vi "Get Focus.vi"(8 "error in":errorcluster, 10 "Start Z":dbl, 11 "CameraTool Class In":refnum<class "CameraTool Class.lvclass">) -> (0 "error out":errorcluster, 2 "focus height":sgl, 3 "CameraTool Class Out":refnum<class "CameraTool Class.lvclass">)   [LabVIEW 2011, in "CameraTool Class.lvclass"]
doc: "This VI returns the \"variance of laplacians\" measure of image focus."
uses:
  CameraTool Class.lvclass
  Gantry Class/Gantry Class.lvclass
  Vec3d Class/Vec3d Class.lvclass
  gVision/Release/gVision.dll
panel:
  in  "interactive":bool
  out "focus return":i32
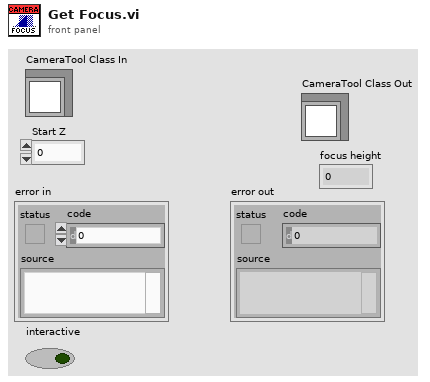
[diagram p1: front panel]
types:
  T1 = enum32{"Map Pixel Pointer", "Unmap Pixel Pointer", "Get Pixels Infos"}
  T2 = typedef "IMAQ Image.ctl" = refnum<image>
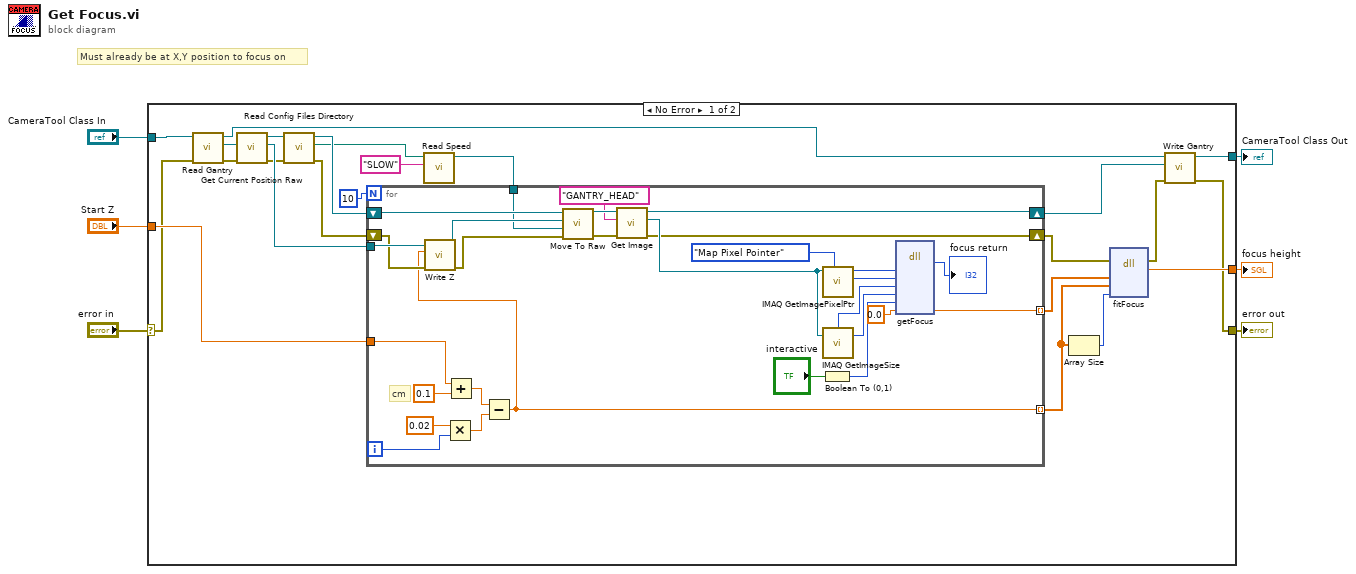
[diagram p0: block diagram]
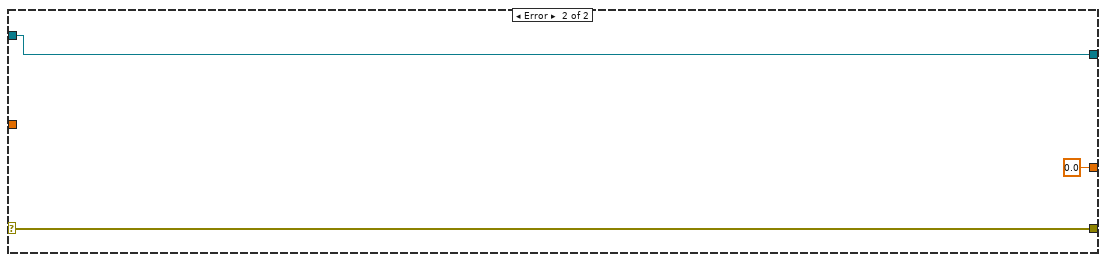
[diagram p2: hidden frame]
diagram:
  # "Must already be at X,Y position to focus on"
  n1 = case shown="No Error" "error in" {
    selector: "error in" -> [w24 w60]
    tunnel: "Start Z" -> [w30 _]
    tunnel: "CameraTool Class In" -> [w29 w62]
    tunnel: [w14 sgl 0.0 ("return type")] -> w3
    tunnel: [w8 w60] -> w2
    tunnel: [w10 w62] -> w1
    frame No Error {
      n2 = call-dynamic "Read Gantry.vi"("error in (no error)"=w24, "Tool Class in"=w29) -> ("error out"=w23:errorcluster, "Gantry Class.lvclass"=w28:refnum<class "Gantry Class.lvclass">, "Tool Class out"=w11:refnum<class "CameraTool Class.lvclass">)  [unwired: 7 in]
      n3 = call "Get Current Position Raw.vi"("error in (no error)"=w23, "Gantry Class in"=w28) -> ("error out"=w22:errorcluster, "Vec3d Class out"=w27:refnum<class "Vec3d Class.lvclass">, "Gantry Class out"=w26:refnum<class "Gantry Class.lvclass">)  [unwired: 7 in]
      n4 = call-dynamic "Read Config Files Directory.vi"("error in (no error)"=w22, "Gantry Class in"=w26) -> ("error out"=w21:errorcluster, "Config Files Directory"=w20:path, "Gantry Class out"=w25:refnum<class "Gantry Class.lvclass">)  [unwired: 7 in]
      n5 = call "Read Speed.vi"("Speeds Label"="SLOW", "Config Files Path"=w20) -> ("Vec3d out"=w18:refnum<class "Vec3d Class.lvclass">)  [unwired: 8 in, 1 out]
      n6 = for {
        N: 10 -> [_]
        tunnel: w30 -> [w50]
        tunnel: w27 -> [w43]
        tunnel: w18 -> [w40]
        tunnel: [w35] -> w17 mode=indexing
        tunnel: [w34] -> w16 mode=indexing
        shift-right: [w33] -> w12
        shift-left: w25 -> [w44]
        shift-right: [w32] -> w13
        shift-left: w21 -> [w41]
        i -> [w48]
        # "cm"
        n7 = Multiply(x=0.02, y=w48) -> (x*y=w45:dbl)
        n8 = Add(x=w50, y=0.1) -> (x+y=w46:dbl)
        n9 = Subtract(x=w46, y=w45) -> (x-y=w34:dbl)
        n10 = call-dynamic "Write Z.vi"("error in (no error)"=w41, "Z"=w34, "Vec3d Class in"=w43) -> ("error out"=w39:errorcluster, "Vec3d Class out"=w42:refnum<class "Vec3d Class.lvclass">)  [unwired: 7 in]
        n11 = call "Move To Raw.vi"("error in (no error)"=w39, "Speed"=w40, "Position"=w42, "Gantry Class in"=w44) -> ("error out"=w37:errorcluster, "Gantry Class out"=w38:refnum<class "Gantry Class.lvclass">)  [unwired: 6 in]
        n12 = call "Get Image.vi"("error in (no error)"=w37, "Camera Name"="GANTRY_HEAD", "Gantry Class in"=w38) -> ("error out"=w32:errorcluster, "Image Out"=w36:T2, "Gantry Class out"=w33:refnum<class "Gantry Class.lvclass">)  [unwired: 6 in]
        n13 = Boolean To (0,1)(Boolean="interactive") -> (0, 1=w52:i16)
        n14 = call "IMAQ GetImagePixelPtr"("Function"=T1."Map Pixel Pointer", "Image"=w36) -> ("LineWidth(Pixels)"=w56:i32, "Pixel Pointer out"=w55:u64)  [unwired: 4 in, 4 out]
        n15 = call "IMAQ GetImageSize"("Image"=w36) -> ("Y Resolution"=w57:i32, "X Resolution"=w58:i32)  [unwired: 3 in, 1 out]
        n16 = dll-call lib="C:/Users/husker/Desktop/gantry/gVision/Release/gVision.dll" fn="getFocus"("img"=w55, "imgLineWidth"=w56, "imgWidth"=w58, "imgHeight"=w57, "interactive"=w52, "focus"=sgl 0.0) -> ("return type"=→"focus return":i32, "focus"=w35:sgl)  [unwired: 8 in, 2 out]
      }
      n17 = Array Size(array=w16) -> (size(s)=w15:i32)
      n18 = dll-call lib="C:/Users/husker/Desktop/gantry/gVision/Release/gVision.dll" fn="fitFocus"(error in=w13, "focus_values"=w17, "heights"=w16, "num_measurements"=w15) -> (error out=w9:errorcluster, "return type"=w14:sgl)  [unwired: 5 in, 1 out]
      n19 = call-dynamic "Write Gantry.vi"("error in (no error)"=w9, "Gantry Class.lvclass"=w12, "Tool Class in"=w11) -> ("error out"=w8:errorcluster, "Tool Class out"=w10:refnum<class "CameraTool Class.lvclass">)  [unwired: 7 in]
    }
    frame Error {
    }
  }
  "CameraTool Class Out" <- w1
  "error out" <- w2
  "focus height" <- w3
